vi "Loss测量.vi"(7 "VISA resource name":refnum<visa-resource-name>, 8 "error in (no error)":errorcluster, 10 "Freq":dbl[](array[numeric]), 11 "RS in":refnum<class "RS.lvclass">) -> (0 "error out":errorcluster, 1 "S12":dbl[](array[numeric]), 2 "S11":dbl[](array[numeric]), 3 "RS out":refnum<class "RS.lvclass">, 4 "S22":dbl[](array[numeric]), 5 "freq":dbl[](array[numeric]), 6 "S21":dbl[](array[numeric]))   [LabVIEW 2015, in "RS.lvclass"]
uses:
  RS.lvclass
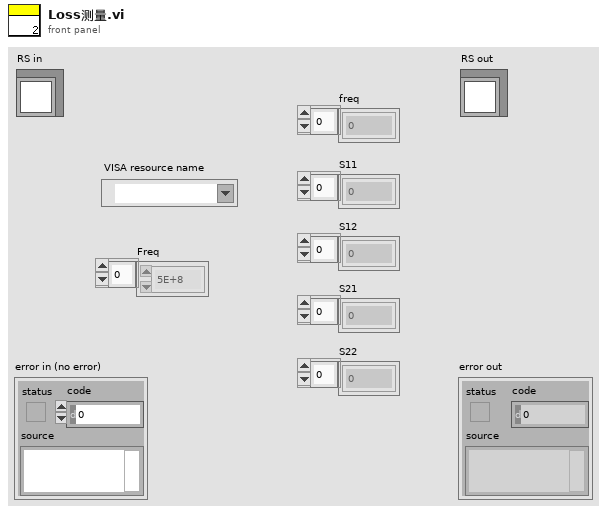
[diagram p1: front panel]
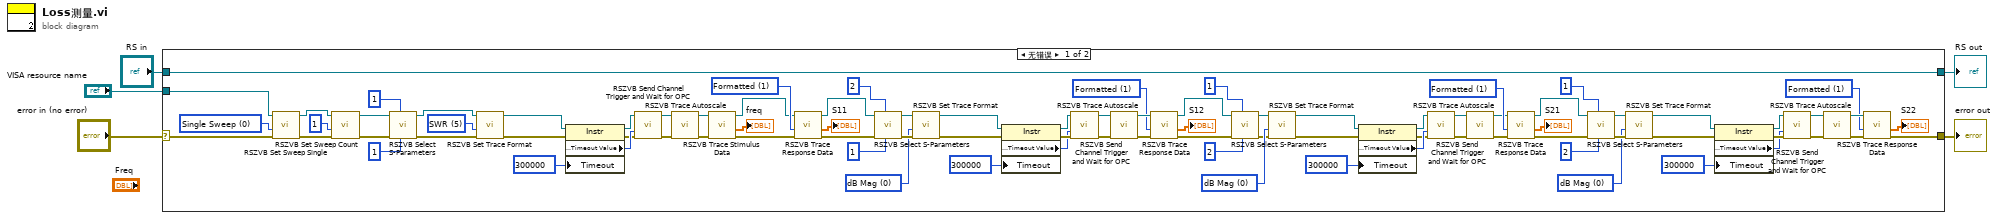
[diagram p0: block diagram]
diagram:
  n1 = case shown="无错误" "error in (no error)" {
    selector: "error in (no error)" -> [w12 w94]
    tunnel: [w6 w94] -> w2
    tunnel: [w92 w93] -> w1
    tunnel: "RS in" -> [w92 w93]
    tunnel: "VISA resource name" -> [w13 _]
    frame No Error {
      w76 = 1 items=["Unformatted", "Formatted", "Unformatted With Trace Mathematics", "Pulse Profile"] ("Data Format (0: Unformatted)")
      w74 = 0 items=["dB Mag", "Phase", "Smith", "Polar", "Delay", "SWR", "Lin Mag", "Real", "Imag", "Inverted Smith", "Unwrapped Phase"] ("Format (0: dB Mag)")
      w69 = 1 items=["Unformatted", "Formatted", "Unformatted With Trace Mathematics", "Pulse Profile"] ("Data Format (0: Unformatted)")
      w71 = 0 items=["dB Mag", "Phase", "Smith", "Polar", "Delay", "SWR", "Lin Mag", "Real", "Imag", "Inverted Smith", "Unwrapped Phase"] ("Format (0: dB Mag)")
      w39 = 1 items=["Unformatted", "Formatted", "Unformatted With Trace Mathematics", "Pulse Profile"] ("Data Format (0: Unformatted)")
      w40 = 0 items=["dB Mag", "Phase", "Smith", "Polar", "Delay", "SWR", "Lin Mag", "Real", "Imag", "Inverted Smith", "Unwrapped Phase"] ("Format (0: dB Mag)")
      w33 = 1 items=["Unformatted", "Formatted", "Unformatted With Trace Mathematics", "Pulse Profile"] ("Data Format (0: Unformatted)")
      w14 = 5 items=["dB Mag", "Phase", "Smith", "Polar", "Delay", "SWR", "Lin Mag", "Real", "Imag", "Inverted Smith", "Unwrapped Phase"] ("Format (0: dB Mag)")
      w30 = 0 items=["Single Sweep", "Continuous Sweep"] ("Single Sweep (1: Continuous Sweep)")
      n2 = call "RSZVB Set Sweep Single.vi"("error in (no error)"=w12, "Single Sweep (1: Continuous Sweep)"=w30, "VISA session"=w13) -> ("error out"=w35:errorcluster, "dup VISA session"=w34:refnum<visa-resource-name>)  [unwired: 7 in]
      n3 = call "RSZVB Set Sweep Count.vi"("error in (no error)"=w35, "Sweep Count (1)"=1, "VISA session"=w34) -> ("error out"=w16:errorcluster, "dup VISA session"=w15:refnum<visa-resource-name>)  [unwired: 7 in]
      n4 = call "RSZVB Select S-Parameters.vi"("Out Port (1)"=1 ("Sweep Count (1)"), "In Port (1)"=1 ("Sweep Count (1)"), "error in (no error)"=w16, "VISA session"=w15) -> ("error out"=w17:errorcluster, "dup VISA session"=w18:refnum<visa-resource-name>)  [unwired: 6 in]
      n5 = call "RSZVB Set Trace Format.vi"("error in (no error)"=w17, "Format (0: dB Mag)"=w14, "VISA session"=w18) -> ("error out"=w20:errorcluster, "dup VISA session"=w19:refnum<visa-resource-name>)  [unwired: 7 in]
      n6 = property class="Instr"(reference=w19, error in=w20, "Timeout"=u32 300000 ("General Settings:Timeout Value")) -> (reference out=w21:refnum<visa-resource-name>, error out=w22:errorcluster, "General Settings:Timeout Value"=w23:u32)
      n7 = call "RSZVB Send Channel Trigger and Wait for OPC.vi"("error in (no error)"=w22, "Timeout (15000)"=w23, "VISA session"=w21) -> ("error out"=w25:errorcluster, "dup VISA session"=w24:refnum<visa-resource-name>)  [unwired: 7 in]
      n8 = call "RSZVB Trace Autoscale.vi"("error in (no error)"=w25, "VISA session"=w24) -> ("error out"=w27:errorcluster, "dup VISA session"=w26:refnum<visa-resource-name>)  [unwired: 8 in]
      n9 = call "RSZVB Trace Stimulus Data.vi"("error in (no error)"=w27, "VISA session"=w26) -> ("error out"=w29:errorcluster, "Trace Data"=→"freq":dbl[], "dup VISA session"=w28:refnum<visa-resource-name>)  [unwired: 7 in]
      n10 = call "RSZVB Trace Response Data.vi"("error in (no error)"=w29, "Data Format (0: Unformatted)"=w33, "VISA session"=w28) -> ("error out"=w55:errorcluster, "Trace Data"=→"S11":dbl[], "dup VISA session"=w54:refnum<visa-resource-name>)  [unwired: 6 in]
      n11 = call "RSZVB Select S-Parameters.vi"("Out Port (1)"=1 ("Sweep Count (1)"), "In Port (1)"=2 ("Sweep Count (1)"), "error in (no error)"=w55, "VISA session"=w54) -> ("error out"=w49:errorcluster, "dup VISA session"=w48:refnum<visa-resource-name>)  [unwired: 6 in]
      n12 = call "RSZVB Set Trace Format.vi"("error in (no error)"=w49, "Format (0: dB Mag)"=w40, "VISA session"=w48) -> ("error out"=w46:errorcluster, "dup VISA session"=w47:refnum<visa-resource-name>)  [unwired: 7 in]
      n13 = property class="Instr"(reference=w47, error in=w46, "Timeout"=u32 300000 ("General Settings:Timeout Value")) -> (reference out=w45:refnum<visa-resource-name>, error out=w44:errorcluster, "General Settings:Timeout Value"=w43:u32)
      n14 = call "RSZVB Send Channel Trigger and Wait for OPC.vi"("error in (no error)"=w44, "Timeout (15000)"=w43, "VISA session"=w45) -> ("error out"=w41:errorcluster, "dup VISA session"=w42:refnum<visa-resource-name>)  [unwired: 7 in]
      n15 = call "RSZVB Trace Autoscale.vi"("error in (no error)"=w41, "VISA session"=w42) -> ("error out"=w53:errorcluster, "dup VISA session"=w52:refnum<visa-resource-name>)  [unwired: 8 in]
      n16 = call "RSZVB Trace Response Data.vi"("error in (no error)"=w53, "Data Format (0: Unformatted)"=w39, "VISA session"=w52) -> ("error out"=w72:errorcluster, "Trace Data"=→"S12":dbl[], "dup VISA session"=w73:refnum<visa-resource-name>)  [unwired: 6 in]
      n17 = call "RSZVB Select S-Parameters.vi"("Out Port (1)"=2 ("Sweep Count (1)"), "In Port (1)"=1 ("Sweep Count (1)"), "error in (no error)"=w72, "VISA session"=w73) -> ("error out"=w60:errorcluster, "dup VISA session"=w61:refnum<visa-resource-name>)  [unwired: 6 in]
      n18 = call "RSZVB Set Trace Format.vi"("error in (no error)"=w60, "Format (0: dB Mag)"=w71, "VISA session"=w61) -> ("error out"=w63:errorcluster, "dup VISA session"=w62:refnum<visa-resource-name>)  [unwired: 7 in]
      n19 = property class="Instr"(reference=w62, error in=w63, "Timeout"=u32 300000 ("General Settings:Timeout Value")) -> (reference out=w64:refnum<visa-resource-name>, error out=w65:errorcluster, "General Settings:Timeout Value"=w66:u32)
      n20 = call "RSZVB Send Channel Trigger and Wait for OPC.vi"("error in (no error)"=w65, "Timeout (15000)"=w66, "VISA session"=w64) -> ("error out"=w68:errorcluster, "dup VISA session"=w67:refnum<visa-resource-name>)  [unwired: 7 in]
      n21 = call "RSZVB Trace Autoscale.vi"("error in (no error)"=w68, "VISA session"=w67) -> ("error out"=w56:errorcluster, "dup VISA session"=w57:refnum<visa-resource-name>)  [unwired: 8 in]
      n22 = call "RSZVB Trace Response Data.vi"("error in (no error)"=w56, "Data Format (0: Unformatted)"=w69, "VISA session"=w57) -> ("error out"=w90:errorcluster, "Trace Data"=→"S21":dbl[], "dup VISA session"=w91:refnum<visa-resource-name>)  [unwired: 6 in]
      n23 = call "RSZVB Select S-Parameters.vi"("Out Port (1)"=2 ("Sweep Count (1)"), "In Port (1)"=1 ("Sweep Count (1)"), "error in (no error)"=w90, "VISA session"=w91) -> ("error out"=w85:errorcluster, "dup VISA session"=w84:refnum<visa-resource-name>)  [unwired: 6 in]
      n24 = call "RSZVB Set Trace Format.vi"("error in (no error)"=w85, "Format (0: dB Mag)"=w74, "VISA session"=w84) -> ("error out"=w82:errorcluster, "dup VISA session"=w83:refnum<visa-resource-name>)  [unwired: 7 in]
      n25 = property class="Instr"(reference=w83, error in=w82, "Timeout"=u32 300000 ("General Settings:Timeout Value")) -> (reference out=w81:refnum<visa-resource-name>, error out=w80:errorcluster, "General Settings:Timeout Value"=w79:u32)
      n26 = call "RSZVB Send Channel Trigger and Wait for OPC.vi"("error in (no error)"=w80, "Timeout (15000)"=w79, "VISA session"=w81) -> ("error out"=w77:errorcluster, "dup VISA session"=w78:refnum<visa-resource-name>)  [unwired: 7 in]
      n27 = call "RSZVB Trace Autoscale.vi"("error in (no error)"=w77, "VISA session"=w78) -> ("error out"=w89:errorcluster, "dup VISA session"=w88:refnum<visa-resource-name>)  [unwired: 8 in]
      n28 = call "RSZVB Trace Response Data.vi"("error in (no error)"=w89, "Data Format (0: Unformatted)"=w76, "VISA session"=w88) -> ("error out"=w6:errorcluster, "Trace Data"=→"S22":dbl[])  [unwired: 6 in, 1 out]
    }
    frame Error {
    }
  }
  "error out" <- w2
  "RS out" <- w1
